vi "FGV CAN.vi"(6 "Aktion":T7, 7 "CAN Data":T1=[{"timestamp"=timestamp(0 s since 1904-01-01), "payload"=[0, 2, 3, 4, 5, 6, 7, 8], "identifier"=2, "type"=0, "extended?"=FALSE, "echo?"=FALSE}, {"timestamp"=timestamp(0 s since 1904-01-01), "payload"=[0, 1, 2, 3, 4, 5, 6, 7], "identifier"=3, "type"=0, "extended?"=FALSE, "echo?"=FALSE}] {"payload" format="%x"; "timestamp" format="%<%.7X\n%x>T"; "type" items=["CAN Data"=0, "CAN Remote"=1, "CAN Bus Error"=2, "CAN 2.0 Data"=8, "CAN FD Data"=16, "CAN FD+BRS Data"=24, "J1939 Data"=192, "Delay"=224, "Log Trigger"=225, "Start Trigger"=226]; "identifier" format="%x"}, 8 "error in (no error)":errorcluster caption="Fehler (Eingang, kein Fehler)", 9 "CAN Messdaten":T4, 10 "Status":u32[](array[numeric]), 11 "Konfig Daten":T5={"Baude Rate"=250000, "COM state"=0, "Frame-ID FTIR Start"=0, "Frame-ID FTIR End"=0, "Frame-ID Status Start"=0, "Frame-ID Status End"=0, "Zustand Information"=0, "Aktion"=0, "Frame-ID FTIR Arry"=[], "Frame-ID Status Arry"=[], "GPS Start"=0, "Interface"="CAN1"} {"Baude Rate" items=["40 kBaud"=40000, "50 kBaud"=50000, "62,5 kBaud"=62500, "80 kBaud"=80000, "83,3 kBaud"=83300, "100 kBaud"=100000, "125 kBaud"=125000, "160 kBaud"=160000, "200 kBaud"=200000, "250 kBaud"=250000, "400 kBaud"=400000, "500 kBaud"=500000, "800 kBaud"=800000, "1 MBaud"=1000000]}) -> (0 "error out":errorcluster caption="Fehler (Ausgang)", 1 "CAN Messdaten":T4, 2 "Status":u32[](array[numeric]), 3 "Konfig Daten":T5={"Baude Rate"=250000, "COM state"=0, "Frame-ID FTIR Start"=0, "Frame-ID FTIR End"=0, "Frame-ID Status Start"=0, "Frame-ID Status End"=0, "Zustand Information"=0, "Aktion"=0, "Frame-ID FTIR Arry"=[], "Frame-ID Status Arry"=[], "GPS Start"=0, "Interface"="CAN1"} {"Baude Rate" items=["40 kBaud"=40000, "50 kBaud"=50000, "62,5 kBaud"=62500, "80 kBaud"=80000, "83,3 kBaud"=83300, "100 kBaud"=100000, "125 kBaud"=125000, "160 kBaud"=160000, "200 kBaud"=200000, "250 kBaud"=250000, "400 kBaud"=400000, "500 kBaud"=500000, "800 kBaud"=800000, "1 MBaud"=1000000]}, 5 "CAN Data":T1=[{"timestamp"=timestamp(0 s since 1904-01-01), "payload"=[0, 2, 3, 4, 5, 6, 7, 8], "identifier"=2, "type"=0, "extended?"=FALSE, "echo?"=FALSE}, {"timestamp"=timestamp(0 s since 1904-01-01), "payload"=[0, 1, 2, 3, 4, 5, 6, 7], "identifier"=3, "type"=0, "extended?"=FALSE, "echo?"=FALSE}] {"payload" format="%x"; "timestamp" format="%<%.7X\n%x>T"; "type" items=["CAN Data"=0, "CAN Remote"=1, "CAN Bus Error"=2, "CAN 2.0 Data"=8, "CAN FD Data"=16, "CAN FD+BRS Data"=24, "J1939 Data"=192, "Delay"=224, "Log Trigger"=225, "Start Trigger"=226]; "identifier" format="%x"})   [LabVIEW 2020, in "CAN Konfig.lvlib"]
uses:
  CAN Konfig.lvlib
  Aktion FGV CAN.ctl
  Konfig Daten PC.ctl
  cRIO/CAN Interface/Baude Rate.ctl
  CAN Messdaten.ctl
  cRIO/CAN Interface/CAN Data.ctl
  <vilib>/xnet/xnet.llb/XNET Frame CAN.ctl
  <vilib>/xnet/xnet.llb/XNET Frame Type CAN.ctl
  Allgemein/allgemeine Sub-VIs.lvlib
  cRIO/CAN Interface/CAN Interface.lvlib
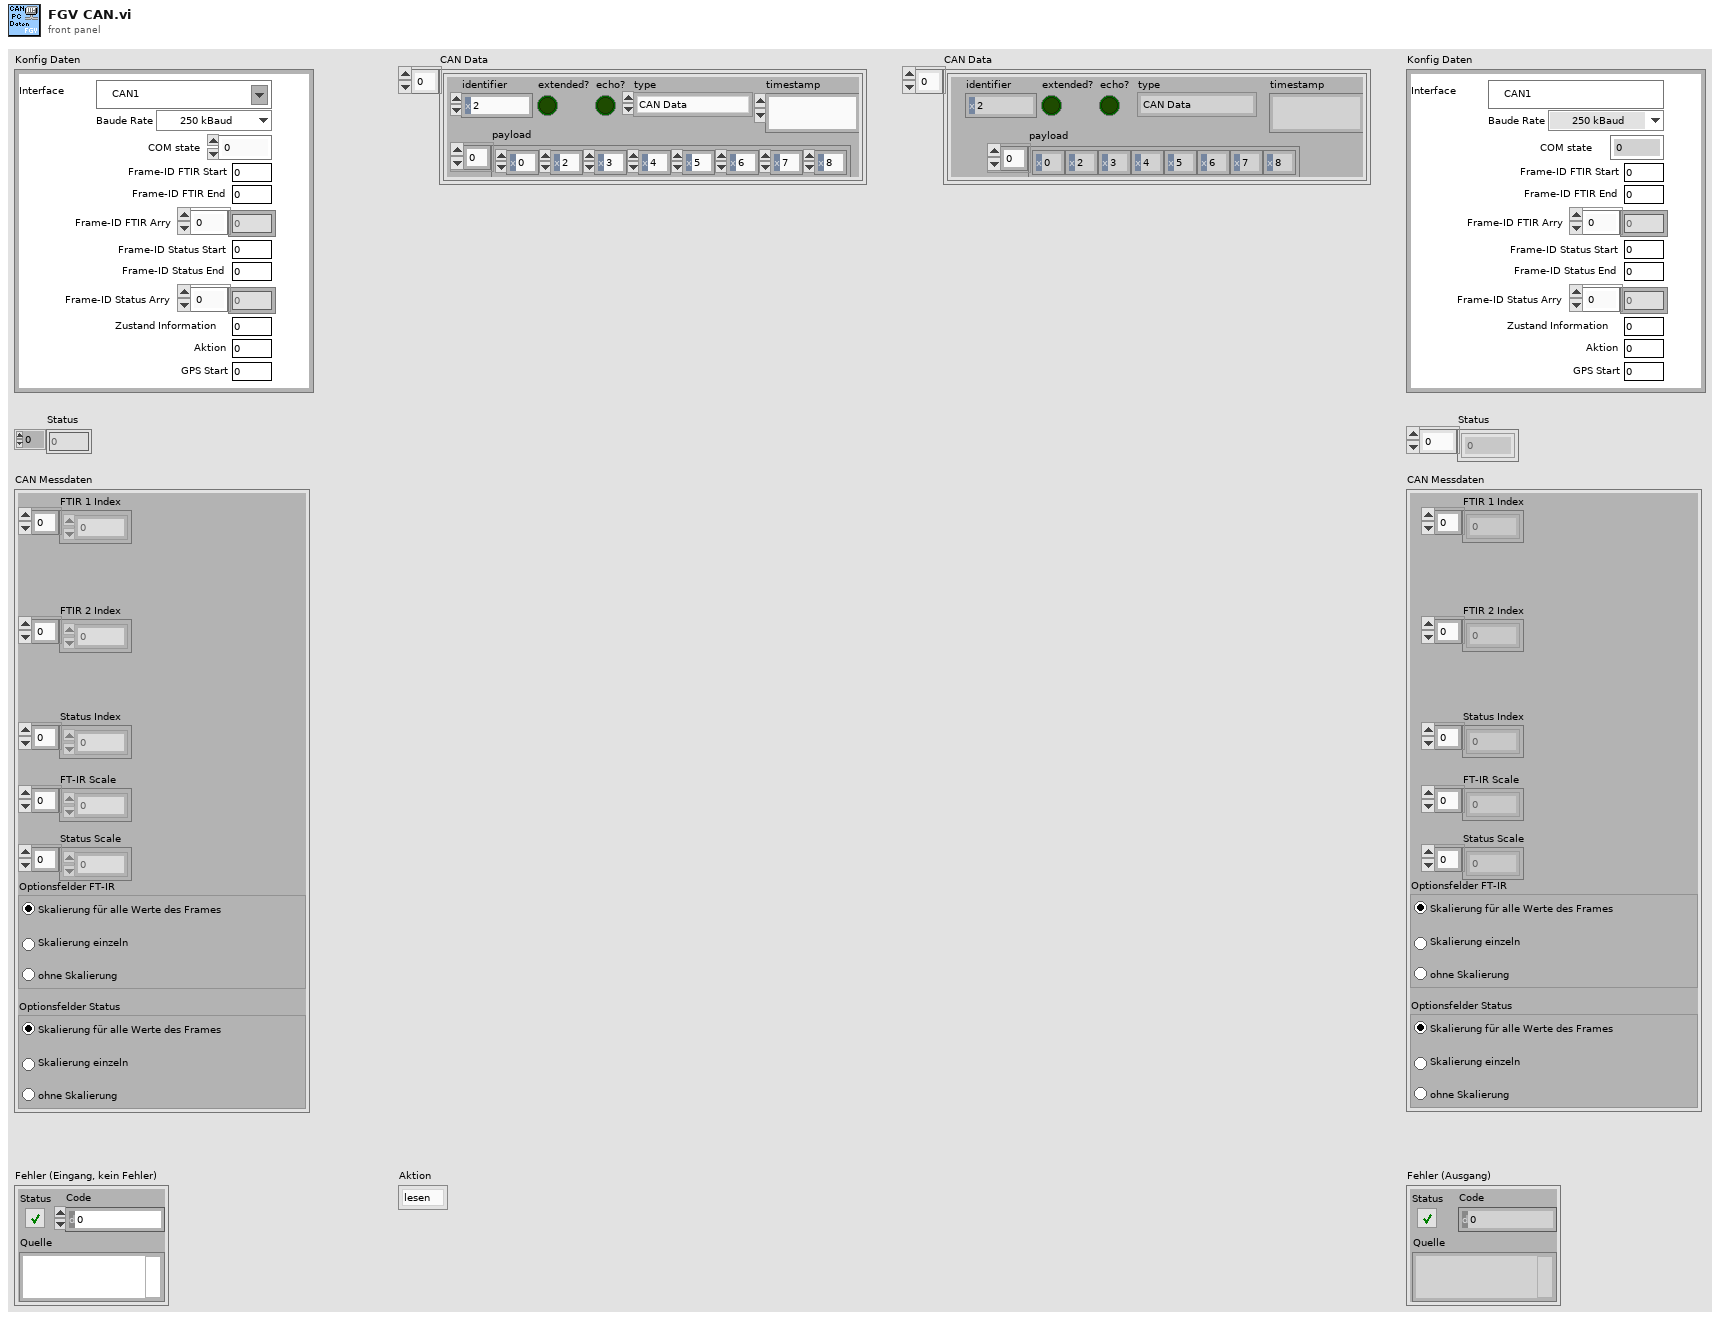
[diagram p1: front panel]
types:
  T1 = typedef "CAN Interface.lvlib/CAN Data.ctl" = T2[]
  T2 = typedef "XNET Frame CAN.ctl" = cluster{"timestamp":timestamp, "payload":u8[], "identifier":u32, "type":T3, "extended?":bool, "echo?":bool}
  T3 = typedef "XNET Frame Type CAN.ctl" = u8
  T4 = typedef "CAN Konfig.lvlib/CAN Messdaten.ctl" = cluster{"FTIR 1 Index":i32[], "FTIR 2 Index":i32[], "Status Index":i32[], "FT-IR Scale":sgl[], "Status Scale":sgl[], "Optionsfelder FT-IR":enum32{"Optionsauswahl 1", "Optionsauswahl 2", "Optionsauswahl 3"}, "Optionsfelder Status":enum32{"Optionsauswahl 1", "Optionsauswahl 2", "Optionsauswahl 3"}}
  T5 = typedef "CAN Konfig.lvlib/Konfig Daten PC.ctl" = cluster{"Baude Rate":T6, "COM state":u8, "Frame-ID FTIR Start":u32, "Frame-ID FTIR End":u32, "Frame-ID Status Start":u32, "Frame-ID Status End":u32, "Zustand Information":u32, "Aktion":u32, "Frame-ID FTIR Arry":u32[], "Frame-ID Status Arry":u32[], "GPS Start":u32, "Interface":refnum<k21>}
  T6 = typedef "CAN Interface.lvlib/Baude Rate.ctl" = u32
  T7 = typedef "CAN Konfig.lvlib/Aktion FGV CAN.ctl" = enum16{"lesen", "schreiben Konfig", "Status", "Messdaten", "laden", "speichern", "CAN Data"}
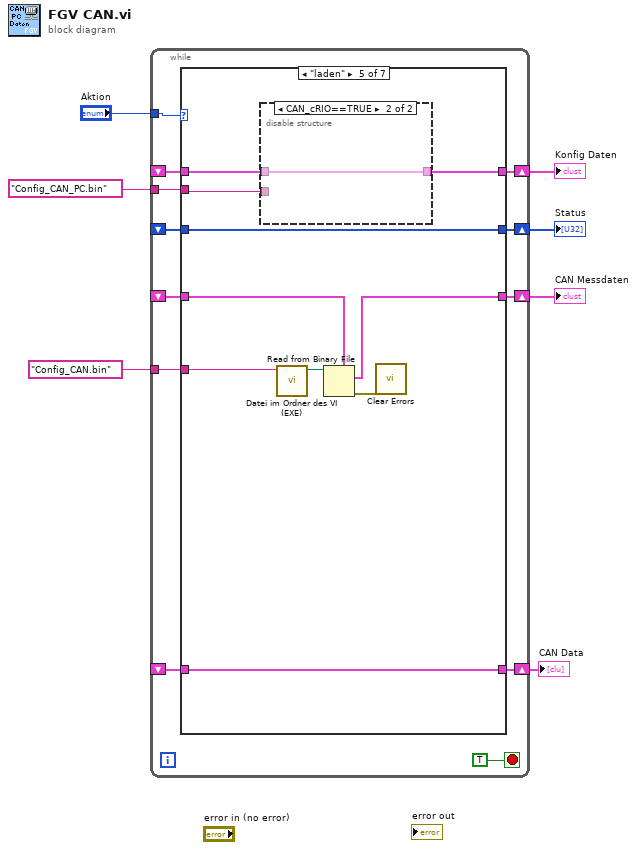
[diagram p0: block diagram]
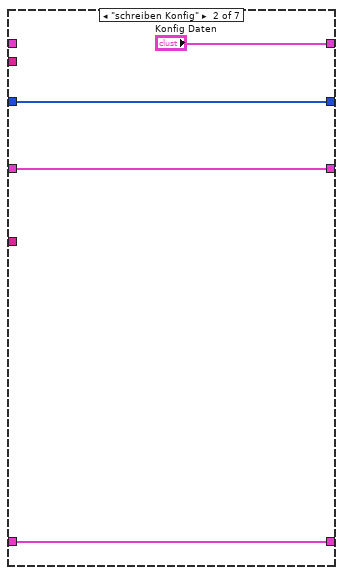
[diagram p3: hidden frame]
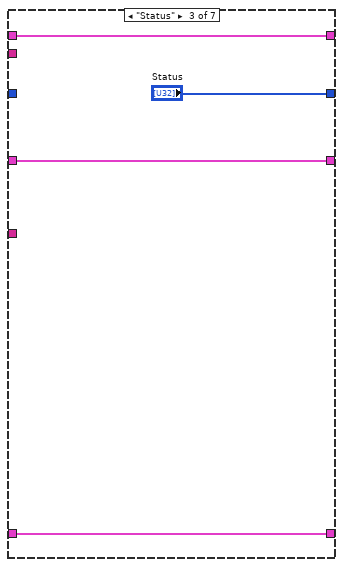
[diagram p4: hidden frame]
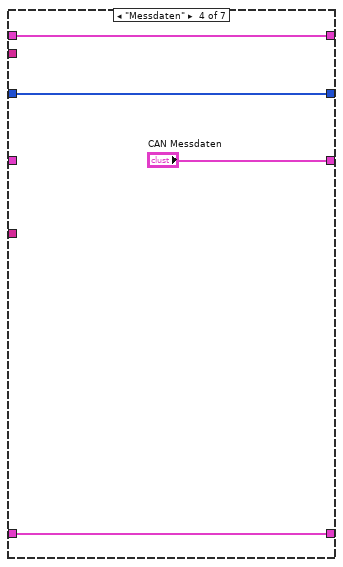
[diagram p5: hidden frame]
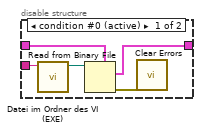
[diagram p6: hidden frame]
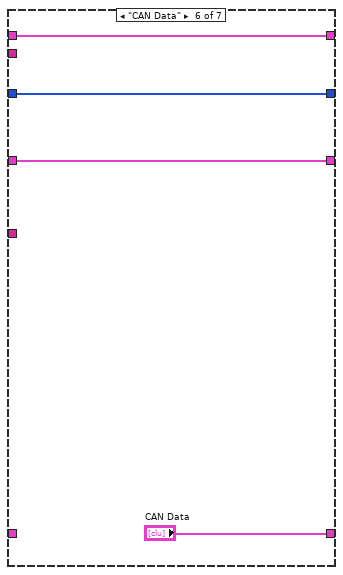
[diagram p7: hidden frame]
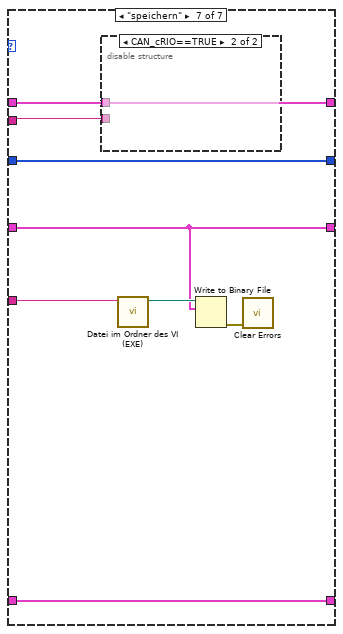
[diagram p8: hidden frame]
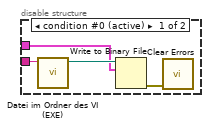
[diagram p9: hidden frame]
diagram:
  n1 = while {
    tunnel: "Aktion" -> [w18]
    shift-right: [w17] -> w6
    shift-left: _ -> [w15]
    shift-right: [w16] -> w5
    shift-left: _ -> [w14]
    shift-right: [w13] -> w4
    shift-left: _ -> [w12]
    tunnel: "Config_CAN.bin" ("Dateiname") -> [w11]
    shift-right: [w10] -> w2
    shift-left: _ -> [w9]
    tunnel: "Config_CAN_PC.bin" ("Dateiname") -> [w8]
    stop <- TRUE stop-if-true
    n2 = case shown="\"laden\"" w18 {
      tunnel: [w20 "Konfig Daten" w28 w32 w36 w52 w57] -> w17
      tunnel: [w23 w27 "Status" w35 w45 w55 w63] -> w16
      tunnel: w15 -> [w20 _ w28 w32 w37 w52 w57]
      tunnel: w14 -> [w23 w27 _ w35 w45 w55 w63]
      tunnel: [w22 w26 w30 "CAN Messdaten" w42 w54 w61] -> w13
      tunnel: w12 -> [w22 w26 w30 _ w41 w54 w61]
      tunnel: w11 -> [_ _ _ _ w44 _ w59]
      tunnel: [w21 w25 w29 w33 w39 "CAN Data" w58] -> w10
      tunnel: w9 -> [w21 w25 w29 w33 w39 _ w58]
      tunnel: w8 -> [_ _ _ _ w38 _ w56]
      frame "lesen", Default {
      }
      frame "schreiben Konfig" {
      }
      frame "Status" {
      }
      frame "Messdaten" {
      }
      frame "laden" {
        n3 = disable-structure shown="CAN_cRIO==TRUE" {
          disable-tunnel: w38 -> [w49 _]
          disable-tunnel: w37 -> [w48 w51]
          disable-tunnel: [w47 w51] -> w36
          frame condition #0 (active) {
            n4 = call "Datei im Ordner des VI (EXE).vi"("Dateiname"=w49) -> ("Dateipfad im Ordner des Haupt-VIs"=w46:path)  [unwired: 8 in, 2 out]
            n5 = Read from Binary File(5:w48, 11:w46) -> (0:w50:errorcluster, 2:w47:T5)  [unwired: 1 in, 5 out]
            n6 = call <vilib>:"Clear Errors.vi"("error in (no error)"=w50) -> ()  [unwired: 5 in, 2 out]
          }
          frame condition #1 {
          }
        }
        n7 = call "Datei im Ordner des VI (EXE).vi"("Dateiname"=w44) -> ("Dateipfad im Ordner des Haupt-VIs"=w43:path)  [unwired: 8 in, 2 out]
        n8 = Read from Binary File(5:w41, 11:w43) -> (0:w40:errorcluster, 2:w42:T4)  [unwired: 1 in, 5 out]
        n9 = call <vilib>:"Clear Errors.vi"("error in (no error)"=w40) -> ()  [unwired: 5 in, 2 out]
      }
      frame "CAN Data" {
      }
      frame "speichern" {
        n10 = disable-structure shown="CAN_cRIO==TRUE" {
          disable-tunnel: w57 -> [w65 _]
          disable-tunnel: w56 -> [w64 _]
          frame condition #0 (active) {
            n11 = call "Datei im Ordner des VI (EXE).vi"("Dateiname"=w64) -> ("Dateipfad im Ordner des Haupt-VIs"=w66:path)  [unwired: 8 in, 2 out]
            n12 = Write to Binary File(file (use dialog)=w66, data=w65) -> (error out=w67:errorcluster)  [unwired: 1 in, 5 out]
            n13 = call <vilib>:"Clear Errors.vi"("error in (no error)"=w67) -> ()  [unwired: 5 in, 2 out]
          }
          frame condition #1 {
          }
        }
        n14 = call "Datei im Ordner des VI (EXE).vi"("Dateiname"=w59) -> ("Dateipfad im Ordner des Haupt-VIs"=w62:path)  [unwired: 8 in, 2 out]
        n15 = Write to Binary File(file (use dialog)=w62, data=w61) -> (error out=w60:errorcluster)  [unwired: 1 in, 5 out]
        n16 = call <vilib>:"Clear Errors.vi"("error in (no error)"=w60) -> ()  [unwired: 5 in, 2 out]
      }
    }
  }
  "Konfig Daten" <- w6
  "Status" <- w5
  "CAN Messdaten" <- w4
  "CAN Data" <- w2
